vi "sub_main_Nstream.vi"(8 "error in":errorcluster) -> (0 "error out":errorcluster)   [LabVIEW 2019]
uses:
  Ctrl/cmd_common.ctl
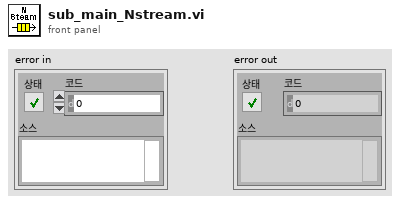
[diagram p1: front panel]
types:
  T1 = typedef "cmd_common.ctl" = enum16{"read", "write"}
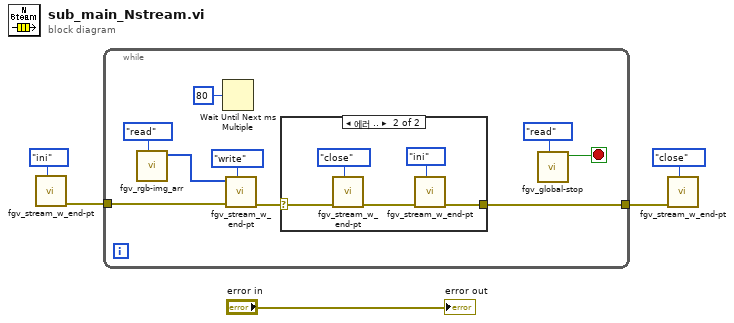
[diagram p0: block diagram]
diagram:
  n1 = call "fgv_stream_w_end-pt.vi"("cmd"=enum16{"ini", "write", "close"}."ini") -> ("error out"=w4:errorcluster)  [unwired: 10 in]
  n2 = while {
    tunnel: w4 -> [w13]
    tunnel: [w11] -> w5
    stop <- w12 stop-if-true
    n3 = call "fgv_rgb-img_arr.vi"("cmd"=cmd_common."read") -> ("rgb_arr"=w8:u8[])  [unwired: 10 in]
    n4 = Wait Until Next ms Multiple(millisecond multiple=u32 80 ("ms 배수")) -> ()  [unwired: 1 out]
    n5 = call "fgv_stream_w_end-pt.vi"("cmd"=enum16{"ini", "write", "close"}."write", "error in"=w13, "rgb_arr"=w8) -> ("error out"=w10:errorcluster)  [unwired: 8 in]
    n6 = case shown="에러 .." w10 {
      selector: w10 -> [w15 w19]
      tunnel: [w15 w17] -> w11
      frame No Error {
      }
      frame Error {
        n7 = call "fgv_stream_w_end-pt.vi"("cmd"=enum16{"ini", "write", "close"}."close", "error in"=w19) -> ("error out"=w18:errorcluster)  [unwired: 9 in]
        n8 = call "fgv_stream_w_end-pt.vi"("cmd"=enum16{"ini", "write", "close"}."ini", "error in"=w18) -> ("error out"=w17:errorcluster)  [unwired: 9 in]
      }
    }
    n9 = call "fgv_global-stop.vi"("cmd"=enum16{"init", "stop", "read"}."read") -> ("val_out"=w12:bool)  [unwired: 10 in]
  }
  n10 = call "fgv_stream_w_end-pt.vi"("cmd"=enum16{"ini", "write", "close"}."close", "error in"=w5) -> ()  [unwired: 9 in, 1 out]
  "error out" <- "error in"
